vi "Command_Spin_Back_Wheels.vi"(3 "Timeout":dbl=3.0, 4 "Speed":dbl, 5 "Startup":bool) -> (0 "Completed":bool=TRUE, 1 "Speed_Out":dbl, 2 "Reinit":bool)   [LabVIEW 2018]
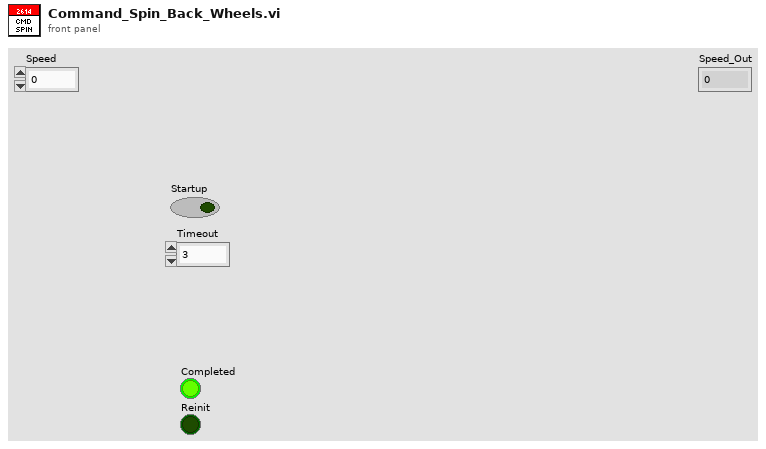
[diagram p1: front panel]
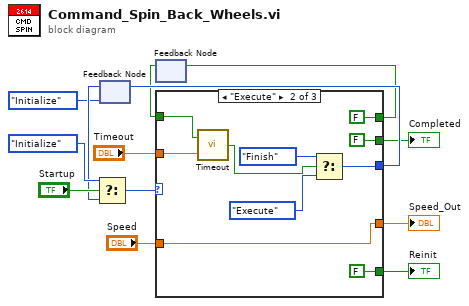
[diagram p0: block diagram]
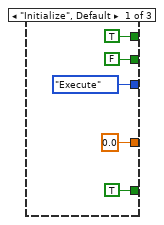
[diagram p2: hidden frame]
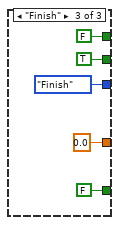
[diagram p3: hidden frame]
diagram:
  n1 = feedback #1(enum16{"Initialize", "Execute", "Finish"}."Initialize" ("f")) -> (w9:enum16{"Initialize", "Execute", "Finish"})
  n2 = Select(t=enum16{"Initialize", "Execute", "Finish"}."Initialize", s="Startup", f=w9) -> (s? t:f=w13:enum16{"Initialize", "Execute", "Finish"})
  n3 = feedback #2() -> (w7:bool)  [unwired: 1 in]
  n4 = case shown="\"Execute\"" w13 {
    tunnel: [enum16{"Initialize", "Execute", "Finish"}."Execute" w25 enum16{"Initialize", "Execute", "Finish"}."Finish" ("f")] -> w10
    tunnel: w7 -> [_ w23 _]
    tunnel: [TRUE FALSE FALSE] -> w8
    tunnel: [FALSE FALSE TRUE] -> w6
    tunnel: [TRUE FALSE FALSE] -> w5
    tunnel: "Timeout" -> [_ w20 _]
    tunnel: [0.0 ("Speed") w19 0.0 ("Speed")] -> w1
    tunnel: "Speed" -> [_ w19 _]
    frame "Initialize", Default {
    }
    frame "Execute" {
      n5 = call "Timeout.vi"("Timeout"=w20, "Initialize"=w23) -> ("Timed Out?"=w21:bool)
      n6 = Select(t=enum16{"Initialize", "Execute", "Finish"}."Finish", s=w21, f=enum16{"Initialize", "Execute", "Finish"}."Execute") -> (s? t:f=w25:enum16{"Initialize", "Execute", "Finish"})
    }
    frame "Finish" {
    }
  }
  "Completed" <- w6
  "Reinit" <- w5
  "Speed_Out" <- w1
  n7 = feedback-in #1(w10) -> ()
  n8 = feedback-in #2(w8) -> ()
